vi "newest map.vi"() -> (1 "newest map":path[](array[path]))   [LabVIEW 2014]
panel:
  out "last mod":timestamp
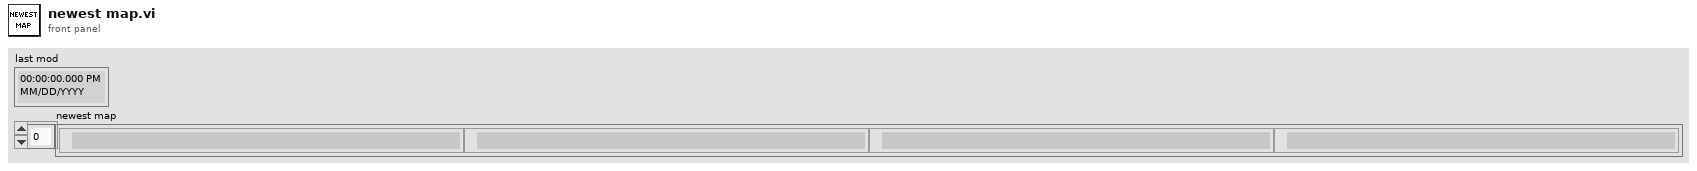
[diagram p1: front panel]
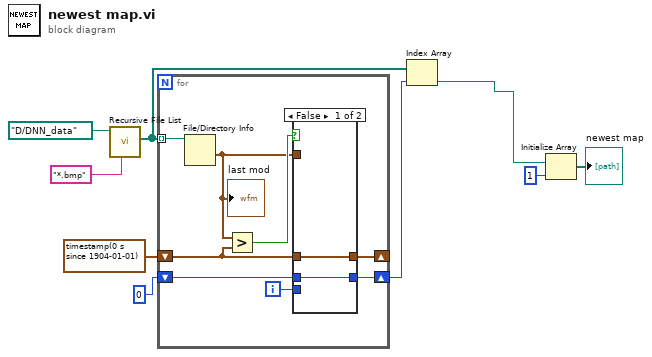
[diagram p0: block diagram]
diagram:
  n1 = call <vilib>:"Recursive File List.vi"("pattern"="*.bmp", "Folder Path"=path "D:/DNN_data" ("path")) -> ("All Files in Dir"=w6:path[])  [unwired: 5 in, 4 out]
  n2 = for {
    tunnel: w6 -> [w17] mode=indexing
    shift-right: [w12] -> _
    shift-left: timestamp(0 s since 1904-01-01) ("last mod") -> [w11]
    shift-right: [w14] -> w5
    shift-left: 0 -> [w10]
    i -> [w15]
    n3 = File/Directory Info(path=w17) -> (last mod=w13:timestamp)  [unwired: 1 in, 6 out]
    "last mod" <- w13
    n4 = Greater?(x=w13, y=w11) -> (0:w16:bool)
    n5 = case shown="False" w16 {
      tunnel: w15 -> [_ w21]
      tunnel: [w18 w21] -> w14
      tunnel: w13 -> [_ w20]
      tunnel: [w19 w20] -> w12
      tunnel: w11 -> [w19 _]
      tunnel: w10 -> [w18 _]
      frame False {
      }
      frame True {
      }
    }
  }
  n6 = Index Array(array=w6, index=w5) -> (element=w2:path)
  n7 = Initialize Array(w2, 1 ("dimension size")) -> (→"newest map":path[])
